vi "configure operation.vi"(7 "Scan Engine configuration":refnum<class "Scan Engine configuration.lvclass">, 8 "error in":errorcluster, 10 "line item in":T2, 11 "engine configuration in":refnum<class "engine configuration.lvclass">) -> (0 "error out":errorcluster, 1 "success":bool, 2 "line item out":T2, 5 "changed":bool)   [LabVIEW 2013, in "Scan Engine editor node.lvclass"]
uses:
  Scan Engine editor node.lvclass
  permissions.ctl
  table line.ctl
  <vilib>/NI/Tag Bus Module Framework/channel/TBM channel.lvclass
  <vilib>/NI/Module Execution Interface/Engine Configuration/engine configuration.lvclass
  <vilib>/NI/TBM Modules/variable/module/configuration/Scan Engine configuration.lvclass
  <vilib>/NI/TBM Modules/variable/module/configuration/url prefix.ctl
  <vilib>/NI/Tag Bus Module Framework/root configuration/TBM configuration.lvclass/TBM configuration.ctl
  <vilib>/NI/Tag Bus Module Framework/channel/TBM channel.lvclass/TBM channel.ctl
  <vilib>/NI/Tag Bus/tag/tag descriptor.lvclass/tag descriptor.ctl
  <vilib>/NI/Tag Bus Module Framework/channel/Read channel classification.vi
  <vilib>/NI/Tag Bus/tag/read data type.vi
  <vilib>/NI/Tag Bus/tag/write tag name.vi
  <vilib>/NI/Tag Bus/tag/write data type.vi
  <vilib>/NI/Tag Bus Module Framework/channel/Write channel classification.vi
  <vilib>/NI/Tag Bus Module Framework/root configuration/Read instance name.vi
  <vilib>/NI/Tag Bus Module Framework/root configuration/create GUID.vi
  <vilib>/NI/Tag Bus/tag/tag descriptor.lvclass
panel:
  in  "Tag":i32(listbox)
  in  "Data Type":i32(listbox)
  in  "hostname":string="localhost"
  in  "Protocol":T1
  in  "Variable Name":string
  in  "cancel":bool
  in  "ok":bool
  in  "Access Type":T3
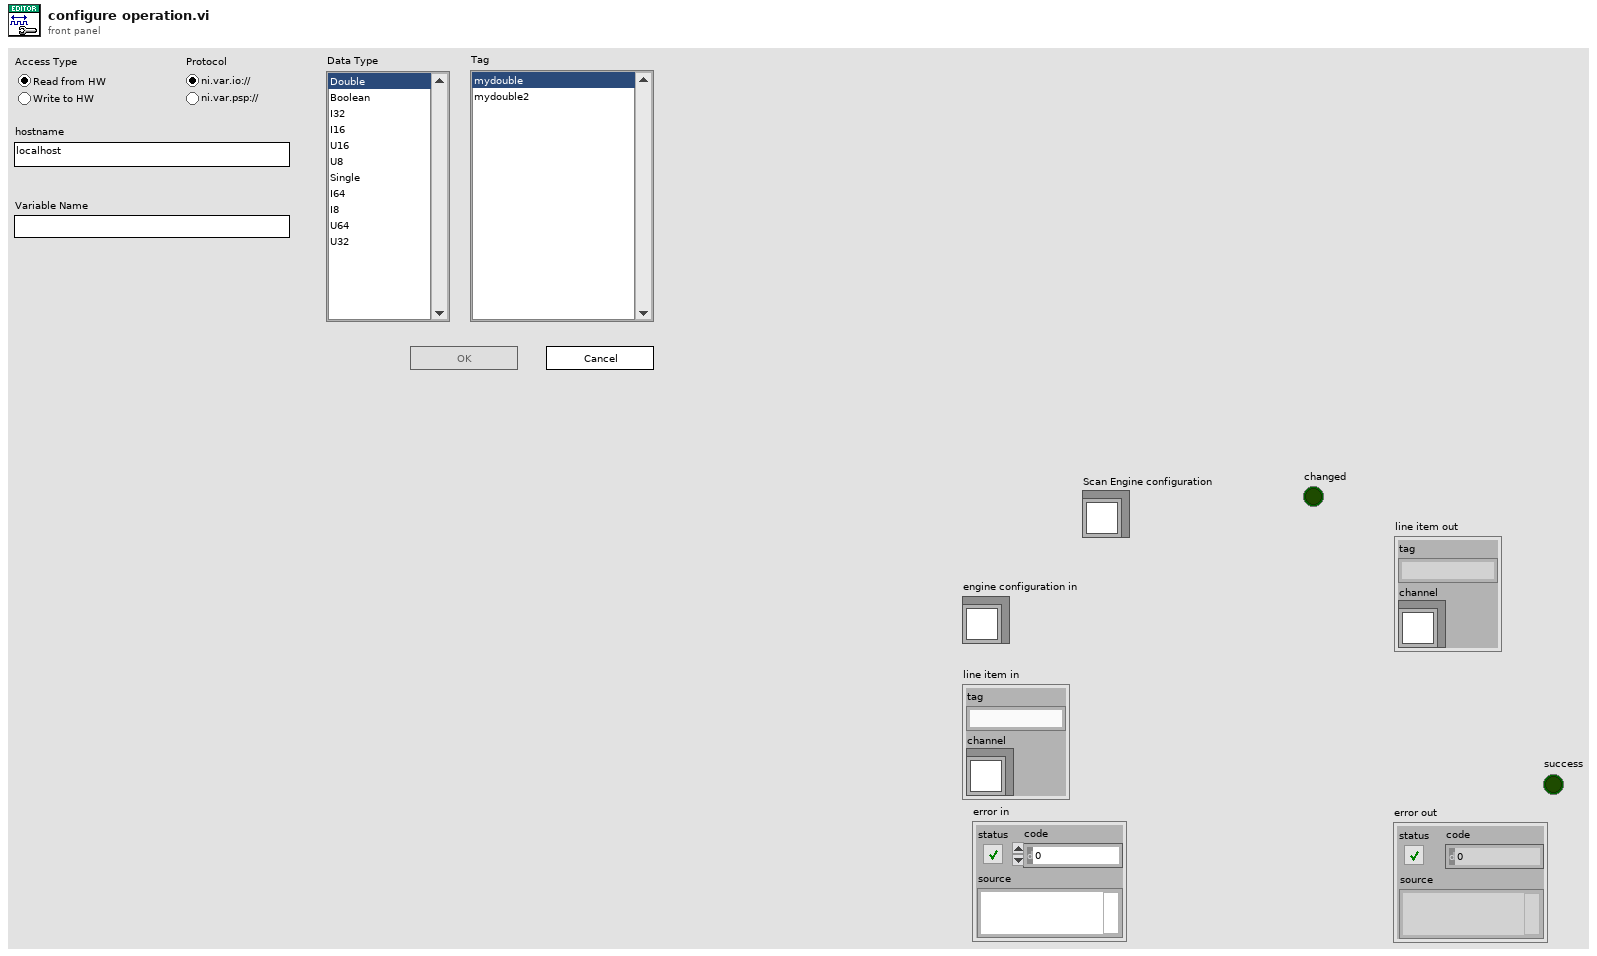
[diagram p1: front panel]
types:
  T1 = typedef "Scan Engine configuration.lvclass/url prefix.ctl" = enum32{"ni.var.io://", "ni.var.psp://"}
  T2 = typedef "Scan Engine editor node.lvclass/table line.ctl" = cluster{"tag":string, "channel":refnum<class "TBM channel.lvclass">}
  T3 = typedef "Scan Engine editor node.lvclass/permissions.ctl" = enum32{"Read from HW", "Write to HW"}
  T4 = typedef "TBM channel.lvclass/channel classification.ctl" = enum16{"input data", "output data", "processing parameter", "processing result"}
  T5 = typedef "tag bus.lvlib/tag descriptor.lvclass/Data Type.ctl" = enum16{"Double", "Single", "I64", "I32", "I16", "I8", "U64", "U32", "U16", "U8", "Boolean", "String", "Array of Double", "Array of Single", "Array of I64", "Array of I32", "Array of I16", "Array of I8", "Array of U64", "Array of U32", "Array of U16", "Array of U8", "Array of Boolean", "Array of String"}
  T6 = enum8{"Enabled", "Disabled", "Disabled and Grayed Out"}
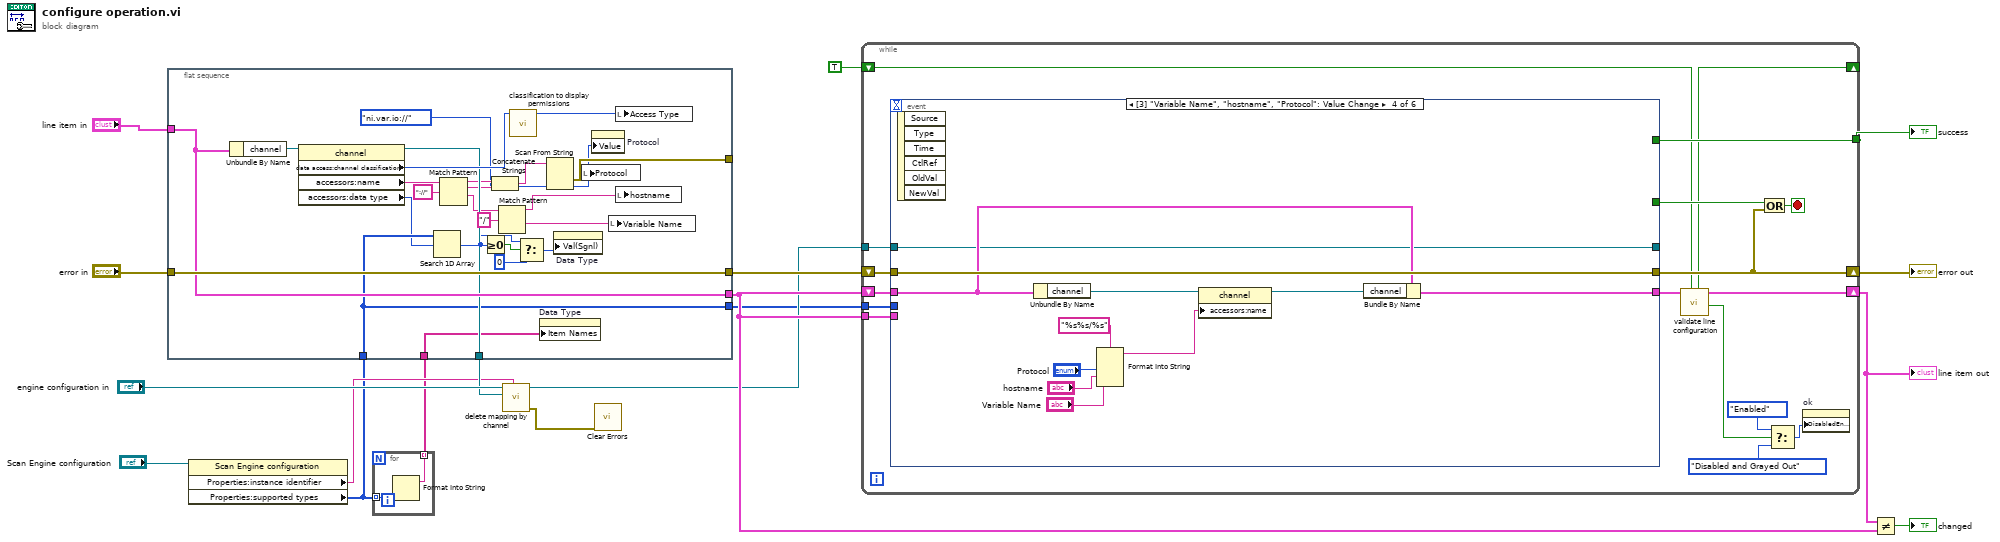
[diagram p0: block diagram]
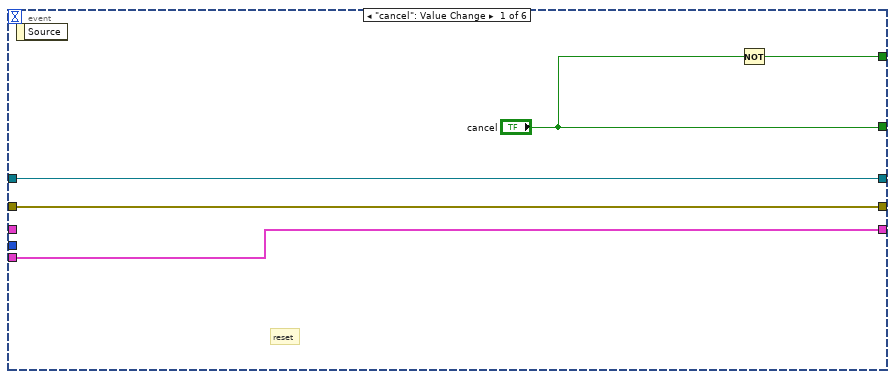
[diagram p2: hidden frame]
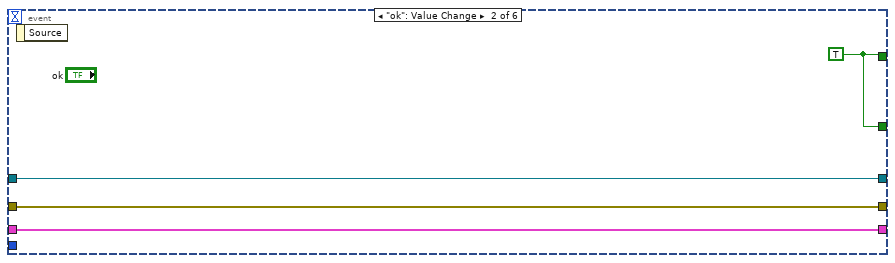
[diagram p3: hidden frame]
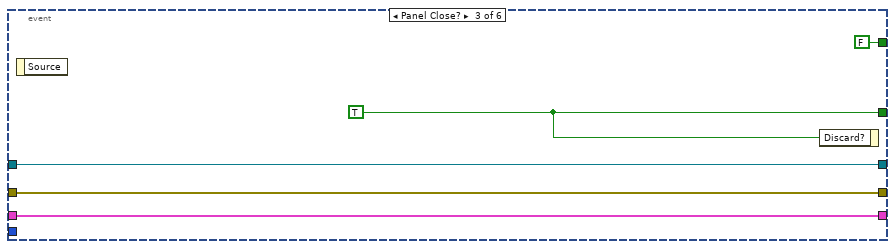
[diagram p4: hidden frame]
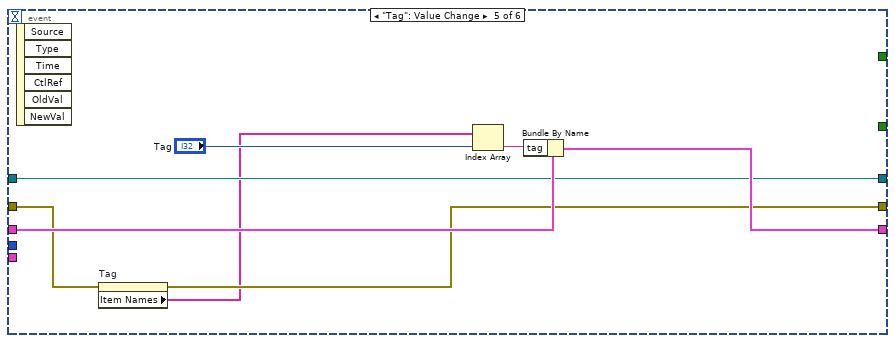
[diagram p5: hidden frame]
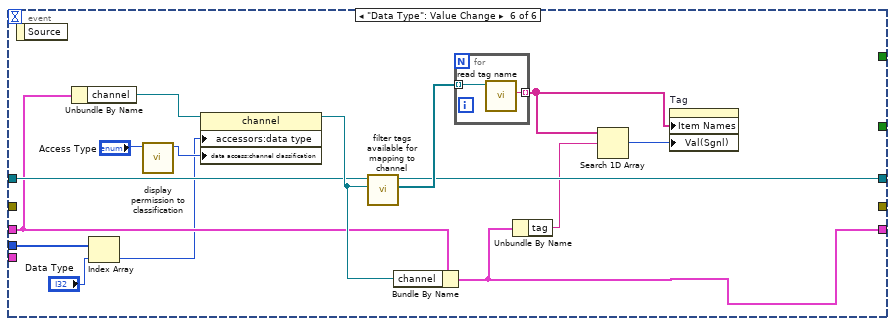
[diagram p6: hidden frame]
diagram:
  n1 = flat-sequence {
    tunnel: [w43] -> w17
    tunnel: "error in" -> [w43]
    tunnel: "line item in" -> [w41]
    tunnel: [w41] -> w11
    tunnel: [w38] -> w8
    tunnel: [w27] -> _
    tunnel: w4 -> [w26]
    tunnel: [w25] -> w3
    tunnel: w2 -> [w25]
    frame #0 {
      n2 = Unbundle By Name(w41) -> ("channel"=w40:refnum<class "TBM channel.lvclass">)
      n3 = property class="channel"(reference=w40) -> (reference out=w38:refnum<class "TBM channel.lvclass">, "data access:channel classification"=w39:T4, "accessors:name"=w37:string, "accessors:data type"=w24:T5)  [unwired: 1 in, 1 out]
      n4 = Search 1D Array(1D array=w25, element=w24) -> (index of element=w22:i32)  [unwired: 1 in]
      n5 = Match Pattern(string=w37, regular expression="://") -> (before substring=w30:string, match substring=w31:string, after substring=w35:string)  [unwired: 1 in, 1 out]
      n6 = Greater Or Equal To 0?(x=w22) -> (x >= 0?=w23:bool)
      n7 = Concatenate Strings(w30, w31) -> (w29:string)
      n8 = Match Pattern(string=w35, regular expression="/") -> (before substring=w33:string, after substring=w32:string)  [unwired: 1 in, 2 out]
      n9 = call "classification to display permissions.vi"("channel classification"=w39) -> ("permissions"=w42:T3)  [unwired: 10 in]
      n10 = Select(t=w22, s=w23, f=0) -> (s? t:f=w20:i32)
      n11 = property on="Data Type" class="LstBox (strict)"("Item Names"=w26) -> ()  [unwired: 2 in, 2 out]
      n12 = Scan From String(input string=w29, default 1=url_prefix."ni.var.io://" ("URL")) -> (error out=w27:errorcluster, output 1=w19:T1)  [unwired: 3 in, 2 out]
      n13 = property on="Data Type" class="LstBox (strict)"("Val(Sgnl)"=w20) -> ()  [unwired: 2 in, 2 out]
      n14 = local write "Protocol"(w19) -> ()
      n15 = property on="Protocol" class="RadioBtnsControl (strict)"("Value"=w19) -> ()  [unwired: 2 in, 2 out]
      n16 = local write "Variable Name"(w32) -> ()
      n17 = local write "Access Type"(w42) -> ()
      n18 = local write "hostname"(w33) -> ()
    }
  }
  n19 = property class="Scan Engine configuration"(reference="Scan Engine configuration") -> ("Properties:instance identifier"=w5:string, "Properties:supported types"=w2:T5[])  [unwired: 1 in, 2 out]
  n20 = for {
    tunnel: w2 -> [w45] mode=indexing
    tunnel: [w44] -> w4 mode=indexing
    n21 = Format Into String(w45) -> (resulting string=w44:string)  [unwired: 3 in, 1 out]
  }
  n22 = call <vilib>:"delete mapping by channel.vi"("owner ID"=w5, "channel"=w8, "engine configuration in"="engine configuration in") -> ("error out"=w7:errorcluster, "engine configuration out"=w9:refnum<class "engine configuration.lvclass">)  [unwired: 7 in]
  n23 = call <vilib>:"Clear Errors.vi"("error in (no error)"=w7) -> ()  [unwired: 6 in, 1 out]
  n24 = while {
    shift-right: [w59] -> w15
    shift-left: w17 -> [w62]
    tunnel: [w61] -> w16
    shift-right: [w54] -> w14
    shift-left: w11 -> [w57]
    tunnel: w11 -> [w56]
    tunnel: w9 -> [w49]
    tunnel: w3 -> [w48]
    shift-right: [w46] -> _
    shift-left: TRUE -> [w47]
    stop <- w58 stop-if-true
    n25 = event shown="[3] \"Variable Name\", \"hostname\", \"Protocol\": Value Change" {
      selector: _ -> [_ _ _ _ _ _]
      dyn-events: _ -> [_ _ _ _ _ _]
      timeout: _ -> [_ _ _ _ _ _]
      tunnel: w62 -> [w67 w69 w76 w87 w90 _]
      tunnel: [w67 w69 w76 w87 w89 _] -> w59
      tunnel: [w66 w71 FALSE _ _ _] -> w61
      tunnel: ["cancel" w71 w74 _ _ _] -> w60
      tunnel: w57 -> [_ w70 w73 w85 w95 w104]
      tunnel: [w64 w70 w73 w86 w94 w100] -> w55
      tunnel: w56 -> [w64 _ _ _ _ _]
      tunnel: w49 -> [w63 w68 w72 w82 w92 w106]
      tunnel: [w63 w68 w72 w82 w92 w105] -> _
      tunnel: w48 -> [_ _ _ _ _ w98]
      event "cancel": Value Change {
        # "reset"
        n26 = event-data() -> ()  [unwired: 1 in, 1 out]
        n27 = Not(x="cancel") -> (.not. x?=w66:bool)
      }
      event "ok": Value Change {
        w71 = TRUE
        n28 = event-data() -> ()  [unwired: 1 in, 1 out]
      }
      event Panel Close? {
        w74 = TRUE ("cancel")
        n29 = event-data() -> ()  [unwired: 1 in, 1 out]
        n30 = event-data("Discard?"=w74) -> ()  [unwired: 1 in, 1 out]
      }
      event "Variable Name", "hostname": Value Change {
        n31 = event-data() -> ()  [unwired: 1 in, 6 out]
        n32 = Unbundle By Name(w85) -> ("channel"=w84:refnum<class "TBM channel.lvclass">)
        n33 = Format Into String(format string="%s%s/%s", "Protocol", "hostname", "Variable Name") -> (resulting string=w78:string)  [unwired: 2 in, 1 out]
        n34 = property class="channel"(reference=w84, "accessors:name"=w78) -> (reference out=w83:refnum<class "TBM channel.lvclass">)  [unwired: 1 in, 1 out]
        n35 = Bundle By Name(cluster=w85, "channel"=w83) -> (w86:T2)
      }
      event "Tag": Value Change {
        n36 = event-data() -> ()  [unwired: 1 in, 6 out]
        n37 = property on="Tag" class="LstBox (strict)"(error in=w90) -> (error out=w89:errorcluster, "Item Names"=w88:string[])  [unwired: 1 in, 1 out]
        n38 = Index Array(array=w88, index="Tag") -> (element=w93:string)
        n39 = Bundle By Name(cluster=w95, "tag"=w93) -> (w94:T2)
      }
      event "Data Type": Value Change {
        n40 = event-data() -> ()  [unwired: 1 in, 1 out]
        n41 = Unbundle By Name(w104) -> ("channel"=w103:refnum<class "TBM channel.lvclass">)
        n42 = Index Array(array=w98, index="Data Type") -> (element=w96:T5)
        n43 = call "display permission to classification.vi"("display permissions"="Access Type") -> ("channel classification"=w107:T4)  [unwired: 10 in]
        n44 = property class="channel"(reference=w103, "accessors:data type"=w96, "data access:channel classification"=w107) -> (reference out=w109:refnum<class "TBM channel.lvclass">)  [unwired: 1 in, 1 out]
        n45 = call <vilib>:"filter tags available for mapping to channel.vi"("channel to map to"=w109, "engine configuration in"=w106) -> ("filtered tags"=w108:refnum<class "tag descriptor.lvclass">[], "engine configuration out"=w105:refnum<class "engine configuration.lvclass">)  [unwired: 8 in]
        n46 = Bundle By Name(cluster=w104, "channel"=w109) -> (w100:T2)
        n47 = for {
          tunnel: w108 -> [w112] mode=indexing
          tunnel: [w111] -> w101 mode=indexing
          n48 = call <vilib>:"read tag name.vi"("system tag in"=w112) -> ("name"=w111:string)  [unwired: 8 in, 2 out]
        }
        n49 = Unbundle By Name(w100) -> ("tag"=w99:string)
        n50 = Search 1D Array(1D array=w101, element=w99) -> (index of element=w102:i32)  [unwired: 1 in]
        n51 = property on="Tag" class="LstBox (strict)"("Item Names"=w101, "Val(Sgnl)"=w102) -> ()  [unwired: 2 in, 2 out]
      }
    }
    n52 = call "validate line configuration.vi"("warn?"=w47, "line in"=w55) -> ("valid?"=w53:bool, "line out"=w54:T2, "still warn?"=w46:bool)  [unwired: 7 in]
    n53 = Compound Arithmetic op=OR(w60, w59) -> (w58:bool)
    n54 = Select(t=T6."Enabled" ("Disabled"), s=w53, f=T6."Disabled and Grayed Out") -> (s? t:f=w50:T6)
    n55 = property on="ok" class="Bool"("DisabledEnum"=w50) -> ()  [unwired: 2 in, 2 out]
  }
  "error out" <- w15
  "success" <- w16
  "line item out" <- w14
  n56 = Not Equal?(x=w14, y=w11) -> (x != y?=→"changed":bool)
